vi "Test_stable_weight.vi"() -> ()   [LabVIEW 2019]
panel:
  out "Double after conversion":dbl
  out "read buffer":string
  in  "VISA resource name":refnum<visa-resource-name>
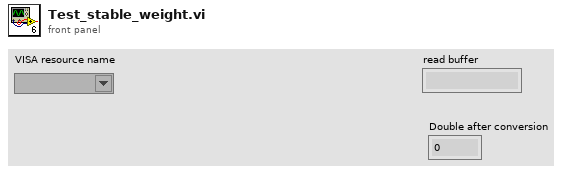
[diagram p1: front panel]
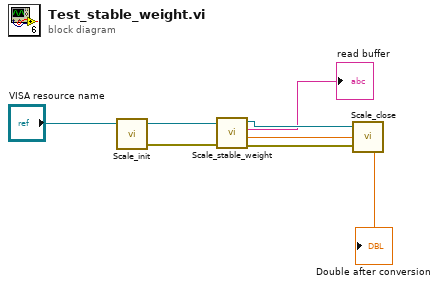
[diagram p0: block diagram]
diagram:
  n1 = call "Scale_init.vi"("VISA resource name\ncheck COM port from \ndevice manager"="VISA resource name") -> ("error out"=w5:errorcluster, "VISA resource name out"=w6:refnum<visa-resource-name>)  [unwired: 3 in]
  n2 = call "Scale_stable_weight.vi"("error in (no error)"=w5, "VISA resource name"=w6) -> ("error out"=w3:errorcluster, "Number after conversion"=→"Double after conversion":dbl, "read buffer"=→"read buffer":string, "VISA resource name out"=w4:refnum<visa-resource-name>)  [unwired: 2 in]
  n3 = call "Scale_close.vi"("error in (no error)"=w3, "VISA resource name"=w4) -> ()  [unwired: 3 in, 1 out]
